vi "Ejercicio2_Estructura Select (versión alternativa).vi"() -> ()   [LabVIEW 2018]
panel:
  in  "stop":bool
  in  "Tanque":dbl(slide) scale=0.0..10.0
  out "Menos de 5":bool
  out "Más de 5":bool
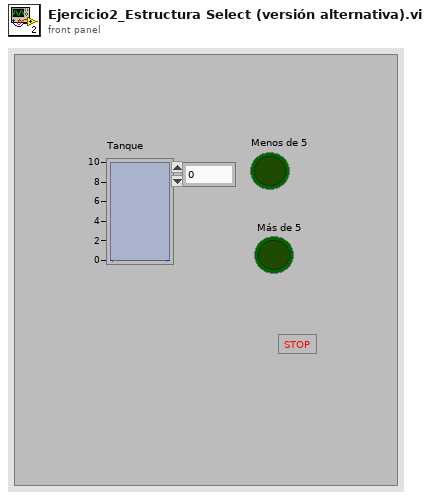
[diagram p1: front panel]
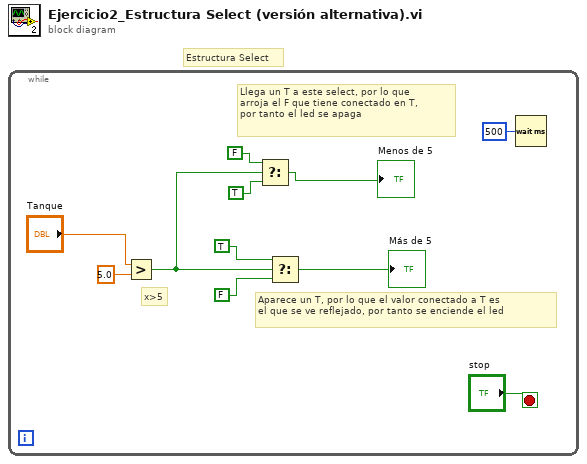
[diagram p0: block diagram]
diagram:
  # "Llega un T a este select, por lo que\narroja el F que tiene conectado en T,\npor tanto el led se apaga"
  # "Estructura Select"
  n1 = while {
    stop <- "stop" stop-if-true
    # "Aparece un T, por lo que el valor conectado a T es\nel que se ve reflejado, por tanto se enciende el led"
    # "x>5"
    n2 = Greater?(x="Tanque", y=5.0) -> (0:w1:bool)
    n3 = Select(t=FALSE, s=w1, f=TRUE) -> (s? t:f=→"Menos de 5":bool)
    n4 = Select(t=TRUE, s=w1, f=FALSE) -> (s? t:f=→"Más de 5":bool)
    n5 = Wait (ms)(milliseconds to wait=u32 500) -> ()  [unwired: 1 out]
  }
